vi "Equation_odd_even_num.vi"() -> ()   [LabVIEW 2026]
panel:
  out "ODD NUMBER":bool
  out "EVEN NUMBER":bool
  out "String":string
  in  "user_input":dbl
  out "O/P: y":dbl
  in  "x":dbl
  # "1.Execute a VI to perform the operation of y=3x+4."
  # "2.operation of checking a given number is odd or \neven"
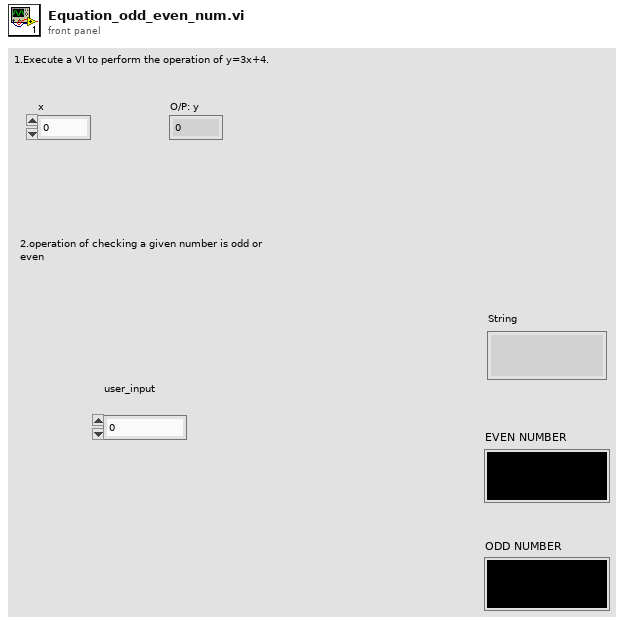
[diagram p1: front panel]
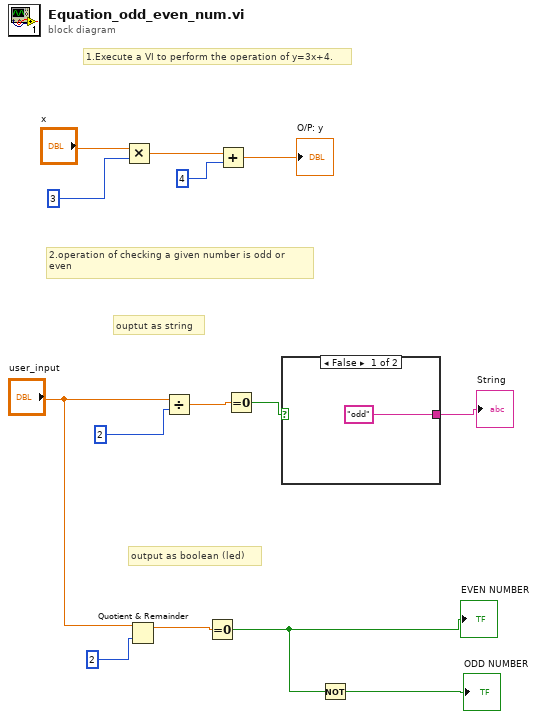
[diagram p0: block diagram]
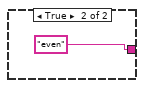
[diagram p2: hidden frame]
diagram:
  # "2.operation of checking a given number is odd or \neven"
  # "1.Execute a VI to perform the operation of y=3x+4."
  # "output as boolean (led)"
  # "ouptut as string"
  n1 = Multiply(x="x", y=3) -> (x*y=w12:dbl)
  n2 = Quotient & Remainder(x="user_input", y=2) -> (x-y*floor(x/y)=w3:dbl)  [unwired: 1 out]
  n3 = Divide(x="user_input", y=2) -> (x/y=w8:dbl)
  n4 = Equal To 0?(x=w3) -> (x = 0?=w2:bool)
  "EVEN NUMBER" <- w2
  n5 = Add(x=w12, y=4) -> (x+y=→"O/P: y":dbl)
  n6 = Equal To 0?(x=w8) -> (x = 0?=w7:bool)
  n7 = case shown="False" w7 {
    tunnel: ["odd" "even"] -> w6
    frame False {
    }
    frame True {
    }
  }
  "String" <- w6
  n8 = Not(x=w2) -> (.not. x?=→"ODD NUMBER":bool)
